vi "Queue Comms Dequeue.vi"(8 "error in (no error)":errorcluster) -> (0 "error out":errorcluster, 3 "Element":T1)   [LabVIEW 2020, in "Wait.lvlib"]
uses:
  Wait.lvlib
  Private Controls/Element.ctl
  Private Controls/Module Action.ctl
  Queue FGV Action.ctl
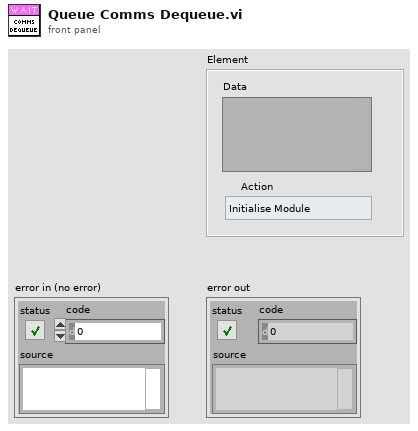
[diagram p1: front panel]
types:
  T1 = typedef "Wait.lvlib/Element.ctl" = cluster{"Action":T2, "Data":variant}
  T2 = typedef "Wait.lvlib/Module Action.ctl" = enum16{"Initialise Module", "Start", "Wait", "Abort", "Error", "Exit"}
  T3 = typedef "Wait.lvlib/Queue FGV Action.ctl" = enum16{"Get", "Set", "Release"}
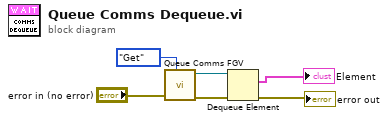
[diagram p0: block diagram]
diagram:
  n1 = call "Queue Comms FGV.vi"("Action"=Queue_FGV_Action."Get", "error in (no error)"="error in (no error)") -> ("error out"=w5:errorcluster, "queue In"=w6:refnum<queue>)  [unwired: 8 in]
  n2 = Dequeue Element(queue=w6, error in (no error)=w5) -> (element=→"Element":T1, error out=→"error out":errorcluster)  [unwired: 1 in, 2 out]
